vi "Start Module.vi"(6 "Show Main VI Diagram on Init (F)":bool, 8 "error in":errorcluster) -> (0 "error out":errorcluster, 1 "Wait for Event Sync?":bool, 2 "Anode Broadcast Events":T1, 3 "Module Was Already Running?":bool, 4 "Module Name":string)   [LabVIEW 2024, in "Anode.lvlib"]
doc: "Launches the Module Main.vi.\n_____\nCreated using DQMH Event Scripter 7.0.1.1316.\n\n<b>Note:</b> This VI was modified by the <b>Validate DQMH Module</b> tool to add calls to the Semaphore VIs to synchronize actions between the Start Module and Stop Module VIs.\n\nThe <b>Validate DQMH Module</b> tool added a 'Module Name' output to this VI."
uses:
  Anode.lvlib
  Broadcast Events--cluster.ctl
  Did Init Argument--cluster.ctl
  Status Updated Argument--cluster.ctl
  Error Reported Argument--cluster.ctl
  Stop Argument--cluster.ctl
  Get Module Execution Status Argument--cluster.ctl
  Broadcast Anode State Argument--cluster.ctl
  Broadcast H2 Sensor Data Argument--cluster.ctl
  <vilib>/Delacor/Delacor QMH/Libraries/Module Admin_class/Delacor_lib_QMH_Module Admin.lvclass
  <vilib>/Delacor/Delacor QMH/Libraries/Module Admin_class/Delacor_lib_QMH_Module Admin.lvclass/Delacor_lib_QMH_Module Admin.ctl
  <vilib>/Delacor/Delacor QMH/Libraries/Module Admin_class/Delacor_lib_QMH_Set External Launch.vi
  <vilib>/Utility/error.llb/Error Cluster From Error Code.vi
  <vilib>/ErrorRing/Error Ring.xnode
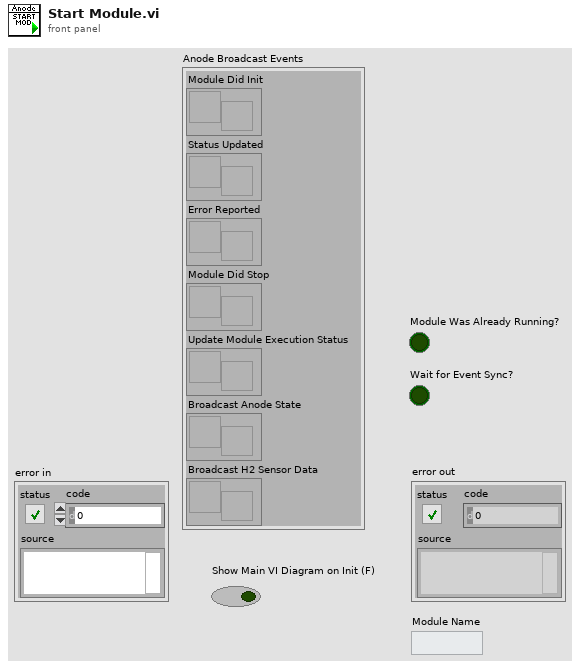
[diagram p1: front panel]
types:
  T1 = typedef "Anode.lvlib/Broadcast Events--cluster.ctl" = cluster{"Module Did Init":refnum<user-event>, "Status Updated":refnum<user-event>, "Error Reported":refnum<user-event>, "Module Did Stop":refnum<user-event>, "Update Module Execution Status":refnum<user-event>, "Broadcast Anode State":refnum<user-event>, "Broadcast H2 Sensor Data":refnum<user-event>}
  T2 = enum32{"Bad", "Idle", "Run top level", "Running"}
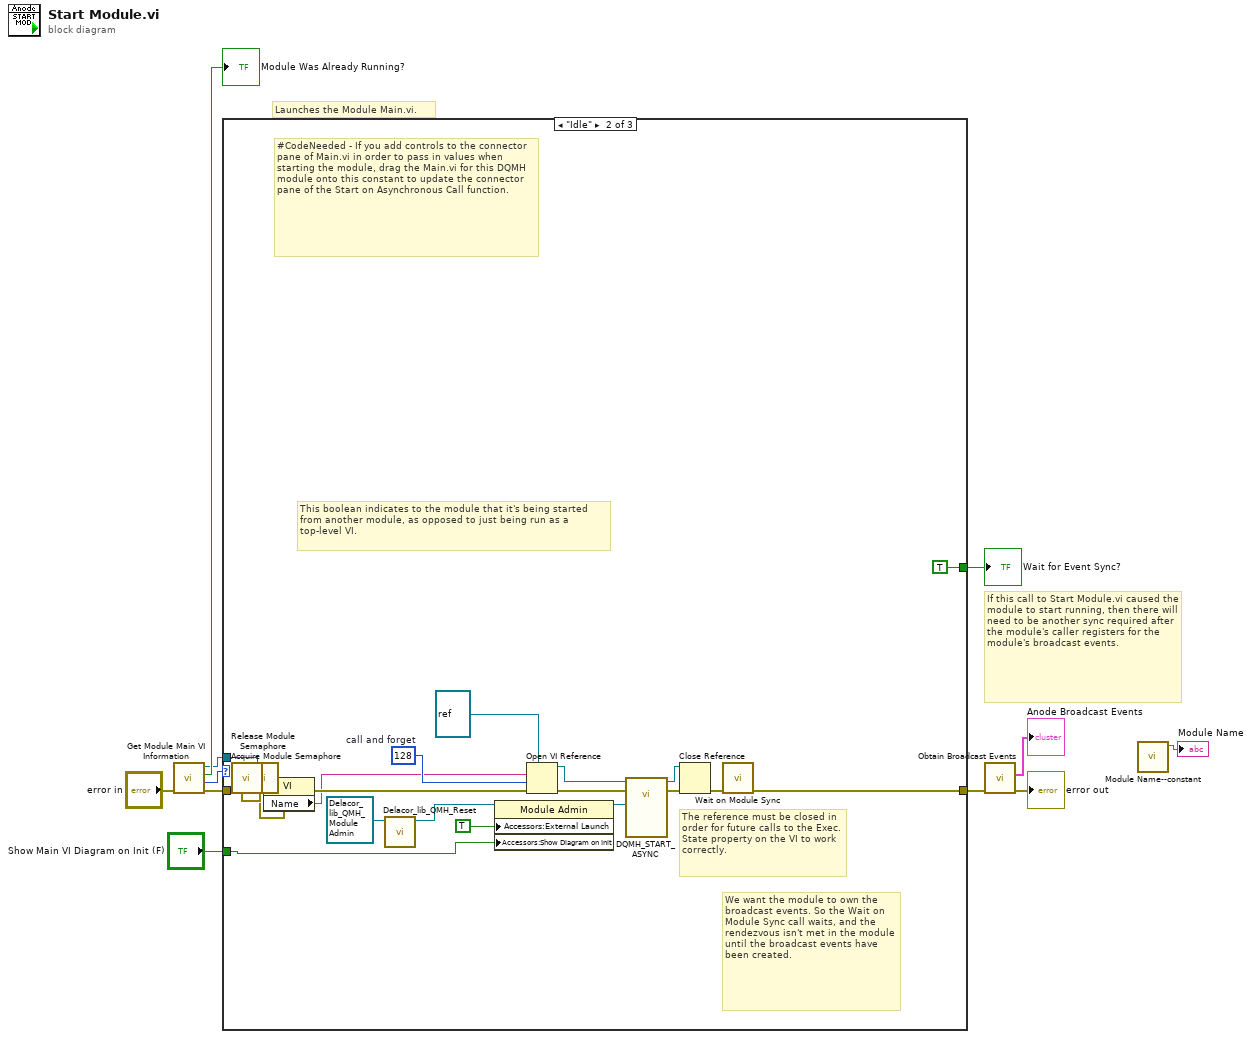
[diagram p0: block diagram]
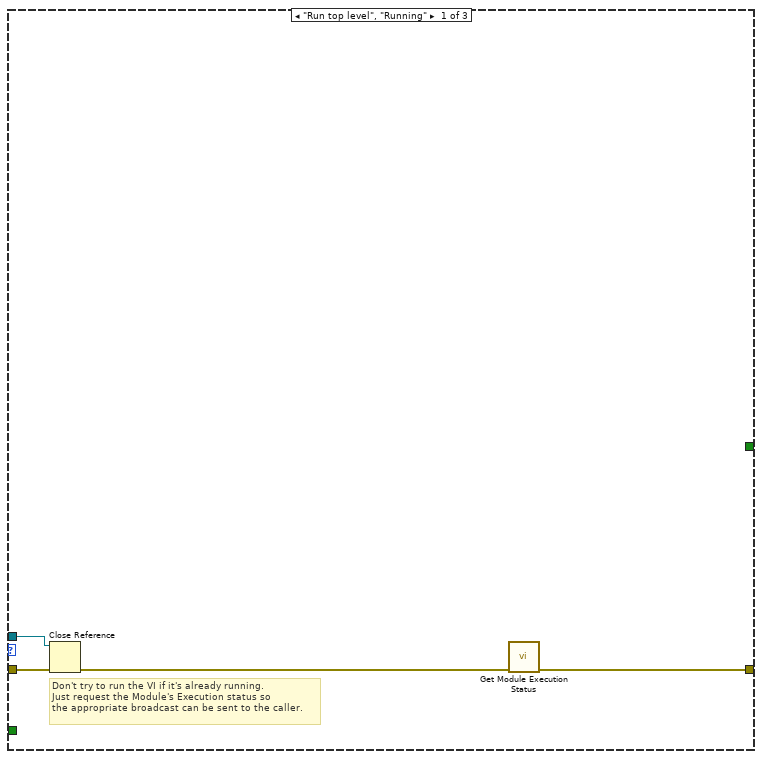
[diagram p2: hidden frame]
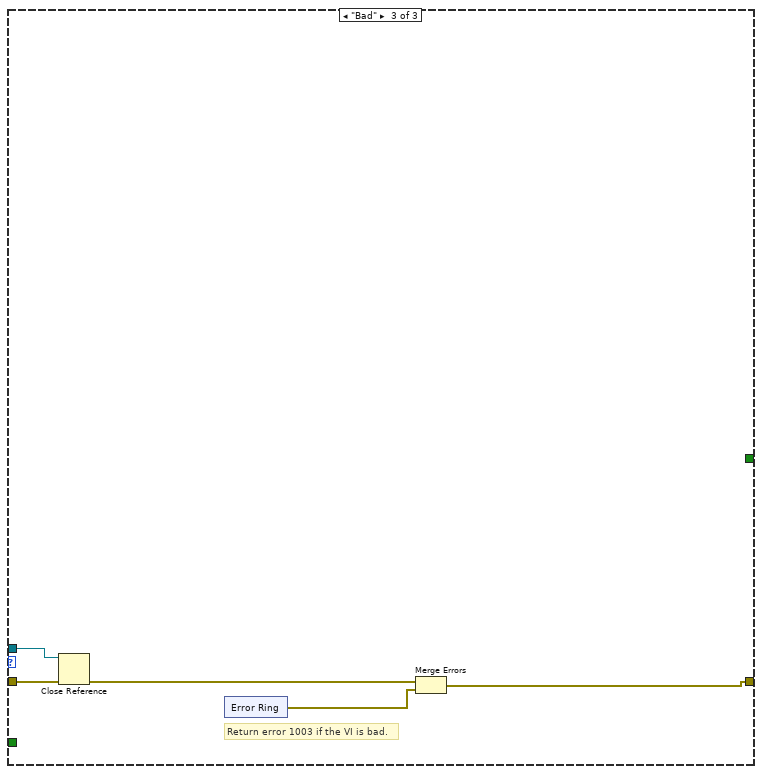
[diagram p3: hidden frame]
diagram:
  # "If this call to Start Module.vi caused the module to start running, then there will need to be another sync required after the module's caller registers for the module's broadcast events."
  # "Launches the Module Main.vi."
  n1 = call "Get Module Main VI Information.vi"("error in (no error)"="error in") -> ("error out"=w9:errorcluster, "Execution State"=w8:T2, "Is Module Running?"=→"Module Was Already Running?":bool, "Module Main VI"=w6:refnum<vi>)  [unwired: 7 in]
  n2 = case shown="\"Idle\"" w8 {
    tunnel: w9 -> [w15 w35 w40]
    tunnel: w6 -> [w14 w30 w39]
    tunnel: [w12 w20 w37] -> w5
    tunnel: [_ TRUE _] -> w11
    tunnel: "Show Main VI Diagram on Init (F)" -> [_ w18 _]
    frame "Run top level", "Running" {
      # "Don't try to run the VI if it's already running.\nJust request the Module's Execution status so\nthe appropriate broadcast can be sent to the caller."
      n3 = Close Reference(reference=w14, error in (no error)=w15) -> (error out=w13:errorcluster)
      n4 = call "Get Module Execution Status.vi"("error in (no error)"=w13) -> ("error out"=w12:errorcluster)  [unwired: 10 in]
    }
    frame "Idle" {
      w27 = 128  # call and forget
      # "#CodeNeeded - If you add controls to the connector pane of Main.vi in order to pass in values when starting the module, drag the Main.vi for this DQMH module onto this constant to update the connector pane of the Start on Asynchronous Call function."
      # "The reference must be closed in order for future calls to the Exec.State property on the VI to work correctly."
      # "We want the module to own the broadcast events. So the Wait on Module Sync call waits, and the rendezvous isn't met in the module until the broadcast events have been created."
      # "This boolean indicates to the module that it's being started from another module, as opposed to just being run as a top-level VI."
      n5 = call "Acquire Module Semaphore.vi"("error in"=w35) -> ("error out"=w17:errorcluster)  [unwired: 10 in]
      n6 = call "Release Module Semaphore.vi"("error in"=w17) -> ("error out"=w16:errorcluster)  [unwired: 10 in]
      n7 = property class="VI"(reference=w30, error in=w16) -> (error out=w29:errorcluster, "Name"=w22:string)  [unwired: 1 out]
      n8 = call-dynamic "Delacor_lib_QMH_Reset.vi"("Mod Admin in"=refnum<class "Delacor_lib_QMH_Module Admin.lvclass"> refnum) -> ("Mod Admin out"=w33:refnum<class "Delacor_lib_QMH_Module Admin.lvclass">)  [unwired: 9 in, 1 out]
      n9 = property on="DQMH_ADMIN_PROP_NODE" class="Module Admin"(reference=w33, "Accessors:External Launch"=TRUE ("DQMH_EXTERNAL_LAUNCH"), "Accessors:Show Diagram on Init"=w18) -> (reference out=w19:refnum<class "Delacor_lib_QMH_Module Admin.lvclass">)  [unwired: 1 in, 1 out]
      n10 = Open VI Reference(type specifier VI Refnum (for type only)=refnum<vi> refnum ("DQMH_TYPE_SPECIFIER"), vi path=w22, options=w27, error in (no error)=w29) -> (vi reference=w25:refnum<vi>, error out=w26:errorcluster)  [unwired: 2 in]
      n11 = call-by-ref "DQMH_START_ASYNC"(reference=w25, error in=w26, "Module Admin"=w19) -> (reference out=w23:refnum<vi>, error out=w24:errorcluster)  [unwired: 11 in]
      n12 = Close Reference ("DQMH_CLOSE_REF")(reference=w23, error in (no error)=w24) -> (error out=w21:errorcluster)
      n13 = call "Wait on Module Sync.vi"("error in (no error)"=w21) -> ("error out"=w20:errorcluster)  [unwired: 10 in]
    }
    frame "Bad" {
      # "Return error 1003 if the VI is bad."
      n14 = Close Reference(reference=w39, error in (no error)=w40) -> (error out=w38:errorcluster)
      n15 = xnode "Error Ring"() -> ("error out"=w36:errorcluster)
      n16 = Merge Errors(w38, w36) -> (w37:errorcluster)
    }
  }
  "Wait for Event Sync?" <- w11
  n17 = call "Obtain Broadcast Events.vi"("error in (no error)"=w5) -> ("error out"=→"error out":errorcluster, "Anode Broadcast Events"=→"Anode Broadcast Events":T1)  [unwired: 9 in]
  n18 = call "Module Name--constant.vi"() -> ("Module Name"=→"Module Name":string)  [unwired: 11 in]
